vi "General Flags.vi"(0 "General Flags In":cluster{"Abort?":bool}, 1 "action":T1=enum."Set Abort Flag", 11 "error in":errorcluster) -> (4 "General Flags Out":cluster{"Abort?":bool}, 15 "error out":errorcluster)   [LabVIEW 2011]
uses:
  General Flags.ctl
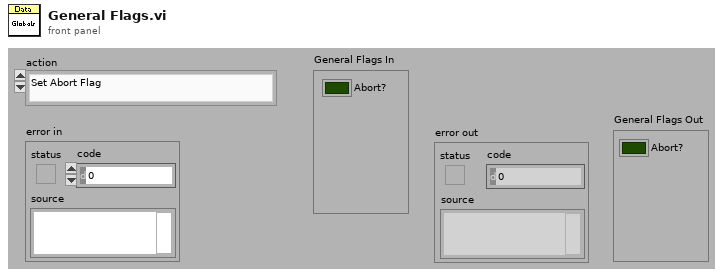
[diagram p1: front panel]
types:
  T1 = typedef "General Flags.ctl" = enum16{"Initialize", "Set Abort Flag", "Get Abort Flag"}
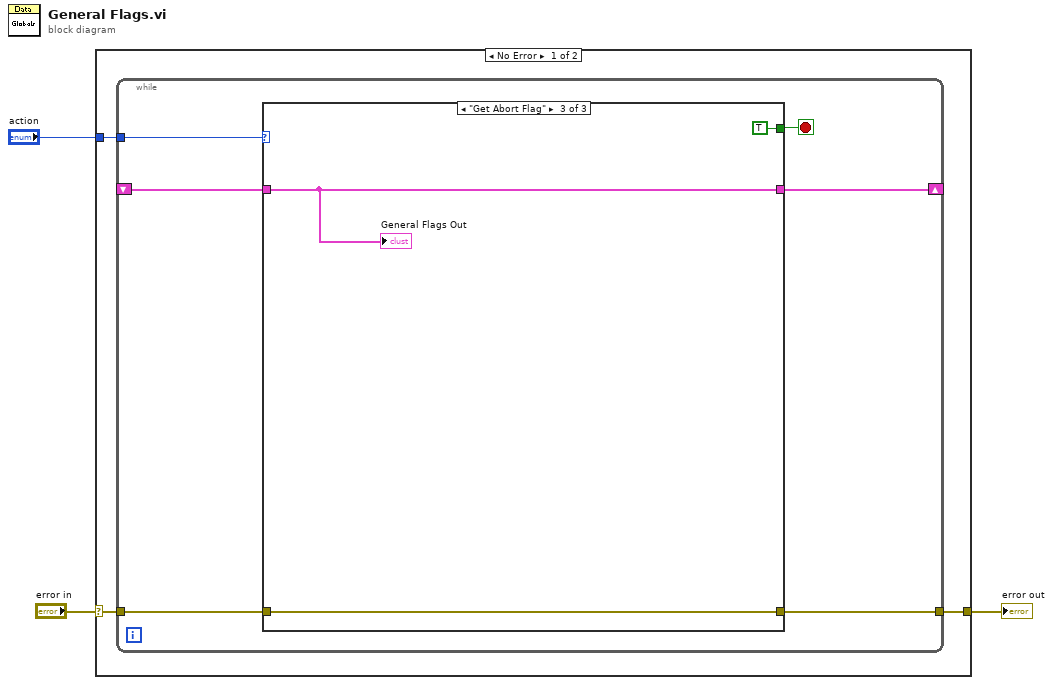
[diagram p0: block diagram]
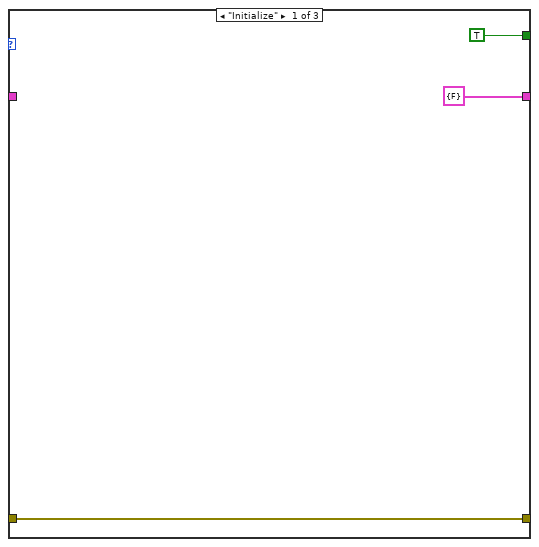
[diagram p2: hidden frame]
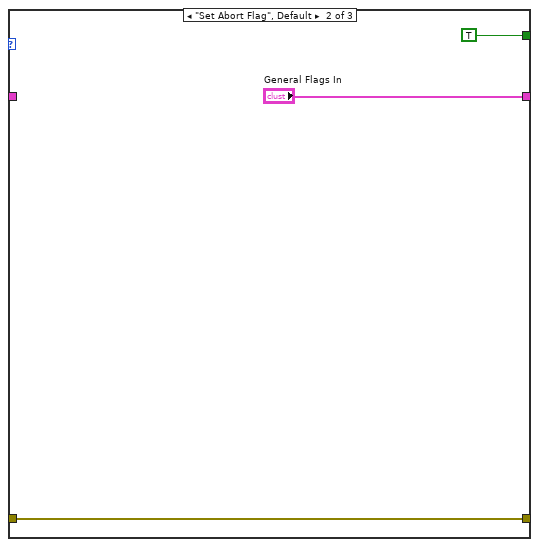
[diagram p3: hidden frame]
diagram:
  n1 = case shown="No Error" "error in" {
    selector: "error in" -> [w6 w22]
    tunnel: [w5 w22] -> w2
    tunnel: "action" -> [w4 _]
    frame No Error {
      n2 = while {
        tunnel: w6 -> [w12]
        tunnel: [w11] -> w5
        tunnel: w4 -> [w9]
        shift-right: [w8] -> _
        shift-left: _ -> [w7]
        stop <- w10 stop-if-true
        n3 = case shown="\"Get Abort Flag\"" w9 {
          tunnel: w12 -> [w13 w17 w19]
          tunnel: [w13 w17 w19] -> w11
          tunnel: [TRUE TRUE TRUE] -> w10
          tunnel: [cluster{"Abort?":bool} {"Abort?"=FALSE} ("General Flags In") "General Flags In" w21] -> w8
          tunnel: w7 -> [_ _ w21]
          frame "Initialize" {
          }
          frame "Set Abort Flag", Default {
          }
          frame "Get Abort Flag" {
            "General Flags Out" <- w21
          }
        }
      }
    }
    frame Error {
    }
  }
  "error out" <- w2
